vi "Detect change of parameters.vi"(10 "AOL_Globals":T1={"Imaging Protocol"=enum."AOL Z-Stack", "Number of POI"=0, "Number of Miniscans"=0, "Number of Trials"=0, "Number of Cycles "=0, "# Averaged Frames"=0, "Laser power (%)"=0, "Pockels (V)"=0.0, "Acquisition Length (sec)"=0.0, "Fill time (us)"=0.0, "POI Dwell time (us)"=0.0, "Miniscan Dwell time per pixel (us)"=0.0, "PMT 1"=0.0, "PMT 2"=0.0, "Back Apperture (mA)"=0.0, "Frame Size"=0, "Center Frequency"=0.0, "Field of View (um)"=175.0, "Field of View (norm)"=0.0, "DwellTime (us)"=0.0, "Ref Dwell Time (us)"=0.0, "Wavelength (nm)"=0.0, "Zoom"=0.0, "AOL Z"=0.0, "AOL Mode"=enum."Raster", "GridXY"=0.0, "GridZ"=0.0, "TriggerPeriod (sec)"=0.0, "Number of Pixels in Miniscan"=0, "Experiment folder path"=path "", "X centre"=0.0, "Y centre"=0.0, "Angle (degrees)"=0.0, "Angle Xs (degrees)"=0.0, "Angle Ys (degrees)"=0.0, "Plane Mode"=0, "Threshold"=[], "Regenerate Chirps"=FALSE, "Rectangle ROI length (pixels)"=0, "Rectangle ROI height (pixels)"=0, "AOD fill"=4900, "StartupDelay"=0, "Samples Wait after Trigger"=5080, "Slip Cycle"=600000, "Add Cycle"=TRUE, "Functional Mode"=enum."Point", "Z Start"=0.0, "Z Stop"=0.0, "# Planes"=0, "Total Pixels"=0, "Variable Miniscan Pixels"=[], "Use Variable Length"=FALSE, "Use Variable Resolution"=FALSE, "Laser power (%) at Z Start"=0, "Laser power (%) at Z Stop"=0, "Ref Z Step"=0} {"Angle Ys (degrees)" format="%#.6g"; "Angle Xs (degrees)" format="%#.6g"; "Plane Mode" items=["XY Plane", "XZ Plane", "YZ Plane", "arbitraryplane"]; "Frame Size" items=["100X100"=100, "128X128"=128, "200X200"=200, "256X256"=256, "512X512"=512, "1024x1024"=1024, "2048x2048"=2048]; "Back Apperture (mA)" format="%#.6g"; "Pockels (V)" format="%#.6g"; "PMT 2" format="%#.6g"; "PMT 1" format="%#.6g"; "Angle (degrees)" format="%#.6g"; "POI Dwell time (us)" format="%#.6g"}, 11 "ZStack":cluster{"Zstart":dbl, "Zstop":dbl, "Zstep":dbl}) -> (3 "Setup has changed":bool)   [LabVIEW 2020]
uses:
  Typedefs/Controls/AOL_Globals.ctl
  Typedefs/Imaging Protocols enum.ctl
  Typedefs/Frame Size.ctl
  Typedefs/AOL modes.ctl
  Typedefs/Plane Mode.ctl
  Typedefs/Functional Mode.ctl
  Typedefs/Chirps regen checked params.ctl
  Global Variables/General Globals.vi
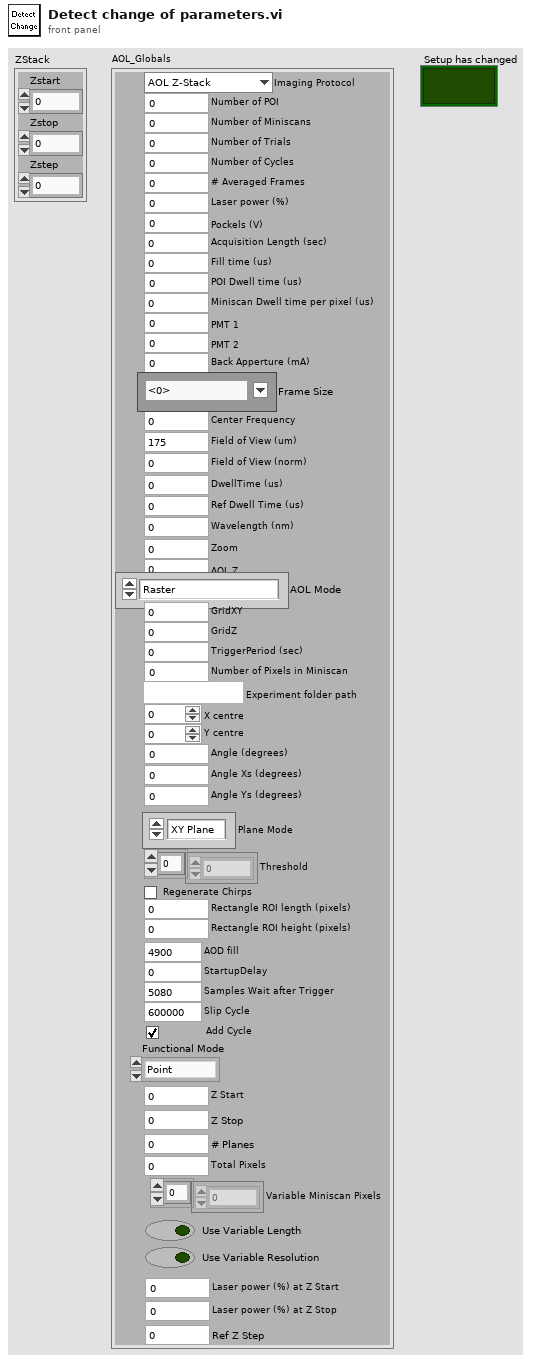
[diagram p1: front panel]
types:
  T1 = typedef "AOL_Globals.ctl" = cluster{"Imaging Protocol":T2, "Number of POI":u16, "Number of Miniscans":u16, "Number of Trials":u16, "Number of Cycles ":u64, "# Averaged Frames":u16, "Laser power (%)":u8, "Pockels (V)":dbl, "Acquisition Length (sec)":dbl, "Fill time (us)":dbl, "POI Dwell time (us)":dbl, "Miniscan Dwell time per pixel (us)":dbl, "PMT 1":dbl, "PMT 2":dbl, "Back Apperture (mA)":dbl, "Frame Size":T3, "Center Frequency":dbl, "Field of View (um)":dbl, "Field of View (norm)":dbl, "DwellTime (us)":dbl, "Ref Dwell Time (us)":dbl, "Wavelength (nm)":dbl, "Zoom":dbl, "AOL Z":dbl, "AOL Mode":T4, "GridXY":dbl, "GridZ":dbl, "TriggerPeriod (sec)":dbl, "Number of Pixels in Miniscan":u16, "Experiment folder path":path, "X centre":dbl, "Y centre":dbl, "Angle (degrees)":dbl, "Angle Xs (degrees)":dbl, "Angle Ys (degrees)":dbl, "Plane Mode":T5, "Threshold":u16[], "Regenerate Chirps":bool, "Rectangle ROI length (pixels)":u16, "Rectangle ROI height (pixels)":u16, "AOD fill":u16, "StartupDelay":i32, "Samples Wait after Trigger":u16, "Slip Cycle":u32, "Add Cycle":bool, "Functional Mode":T6, "Z Start":dbl, "Z Stop":dbl, "# Planes":i32, "Total Pixels":i32, "Variable Miniscan Pixels":u16[], "Use Variable Length":bool, "Use Variable Resolution":bool, "Laser power (%) at Z Start":u8, "Laser power (%) at Z Stop":u8, "Ref Z Step":i8}
  T2 = typedef "Imaging Protocols enum.ctl" = enum16{"AOL Z-Stack", "Motor Z Stack", "Parameter Sweep", "Functional Acquisition", "Single Plane Acquisition", "Volume Acquisition", "Live Imaging", "Live Plane Imaging", "Live Volume Imaging"}
  T3 = typedef "Frame Size.ctl" = u16
  T4 = typedef "AOL modes.ctl" = enum16{"Raster", "Structural", "Pointing", "Mini Scan", "Alignment"}
  T5 = typedef "Plane Mode.ctl" = u16
  T6 = typedef "Functional Mode.ctl" = enum16{"Point", "Line", "Patch", "Plane", "Volume"}
  T7 = typedef "Chirps regen checked params.ctl" = cluster{"Laser power (%)":u8, "Field of View":dbl, "Frame Size":T3, "AOL Z":dbl, "DwellTime (us)":dbl, "Zoom":dbl, "Number of POI":u16, "Number of Miniscans":u16, "POI Dwell time (us)":dbl, "Miniscan Dwell time per pixel (us)":dbl, "Number of Pixels in Miniscan":u16, "X centre":dbl, "Y centre":dbl, "Wavelength (nm)":dbl, "Angle (degrees)":dbl, "Angle Xs (degrees)":dbl, "Angle Ys (degrees)":dbl, "Plane Mode":T5, "Regenerate Chirps":bool, "Ref Z Step":i8}
  T8 = cluster{"ZStack":cluster{"Zstart":dbl, "Zstop":dbl, "Zstep":dbl}, "Checked parameters":T7}
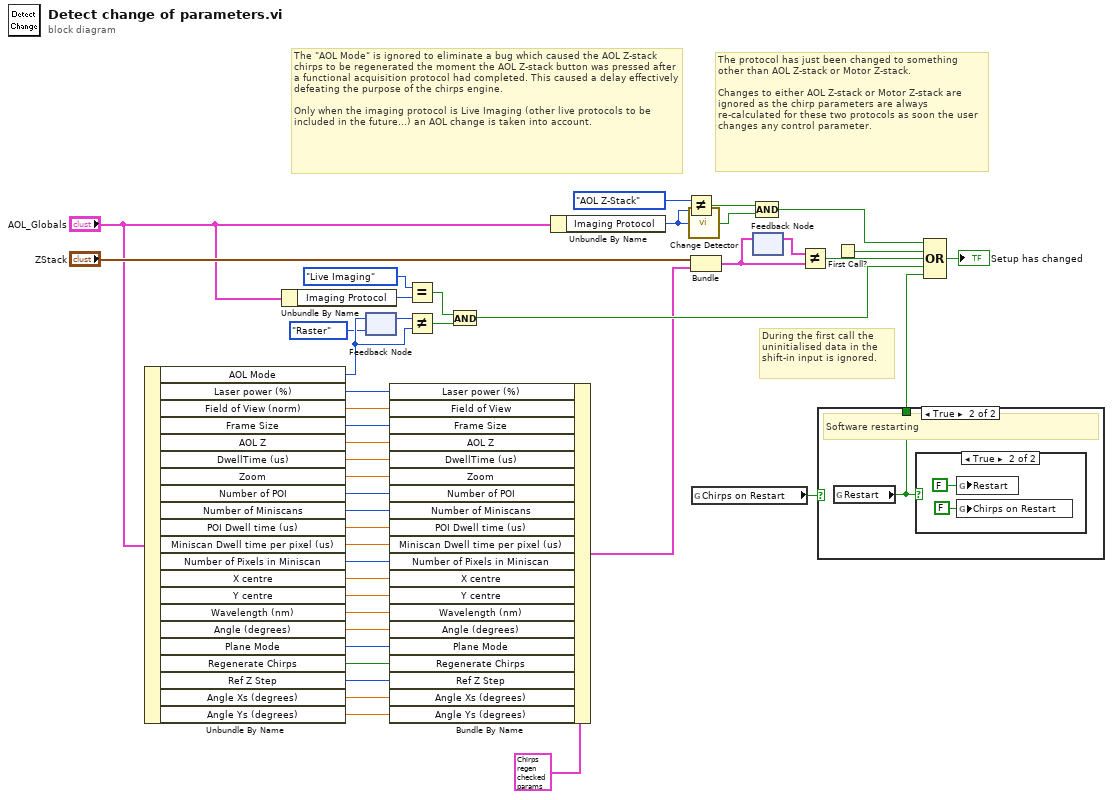
[diagram p0: block diagram]
diagram:
  # "The \"AOL Mode\" is ignored to eliminate a bug which caused the AOL Z-stack chirps to be regenerated the moment the AOL Z-stack button was pressed after a functional acquisition protocol had completed. This caused a delay effectively defeating the purpose of the chirps engine.\n\nOnly when the imaging protocol is Live Imaging (other live protocols to be included in the future...) an AOL change is taken into account."
  # "The protocol has just been changed to something other than AOL Z-stack or Motor Z-stack.\n\nChanges to either AOL Z-stack or Motor Z-stack are ignored as the chirp parameters are always re-calculated for these two protocols as soon the user changes any control parameter."
  # "During the first call the uninitialised data in the shift-in input is ignored."
  n1 = Unbundle By Name("AOL_Globals") -> ("AOL Mode"=w16:T4, "Laser power (%)"=w35:u8, "Field of View (norm)"=w34:dbl, "Frame Size"=w33:T3, "AOL Z"=w32:dbl, "DwellTime (us)"=w31:dbl, "Zoom"=w30:dbl, "Number of POI"=w29:u16, "Number of Miniscans"=w28:u16, "POI Dwell time (us)"=w27:dbl, "Miniscan Dwell time per pixel (us)"=w26:dbl, "Number of Pixels in Miniscan"=w25:u16, "X centre"=w24:dbl, "Y centre"=w23:dbl, "Wavelength (nm)"=w22:dbl, "Angle (degrees)"=w21:dbl, "Plane Mode"=w20:T5, "Regenerate Chirps"=w19:bool, "Ref Z Step"=w3:i8, "Angle Xs (degrees)"=w2:dbl, "Angle Ys (degrees)"=w1:dbl)
  n2 = Unbundle By Name("AOL_Globals") -> ("Imaging Protocol"=w15:T2)
  n3 = feedback-in #1(w16) -> ()
  n4 = feedback #1(AOL_modes."Raster" ("AOL Mode")) -> (w18:T4)
  n5 = Bundle By Name(cluster=T7 {"Laser power (%)"=0, "Field of View"=0.0, "Frame Size"=0, "AOL Z"=0.0, "DwellTime (us)"=0.0, "Zoom"=0.0, "Number of POI"=0, "Number of Miniscans"=0, "POI Dwell time (us)"=0.0, "Miniscan Dwell time per pixel (us)"=0.0, "Number of Pixels in Miniscan"=0, "X centre"=0.0, "Y centre"=0.0, "Wavelength (nm)"=0.0, "Angle (degrees)"=0.0, "Angle Xs (degrees)"=0.0, "Angle Ys (degrees)"=0.0, "Plane Mode"=0, "Regenerate Chirps"=FALSE, "Ref Z Step"=0} ("Checked parameters"), "Laser power (%)"=w35, "Field of View"=w34, "Frame Size"=w33, "AOL Z"=w32, "DwellTime (us)"=w31, "Zoom"=w30, "Number of POI"=w29, "Number of Miniscans"=w28, "POI Dwell time (us)"=w27, "Miniscan Dwell time per pixel (us)"=w26, "Number of Pixels in Miniscan"=w25, "X centre"=w24, "Y centre"=w23, "Wavelength (nm)"=w22, "Angle (degrees)"=w21, "Plane Mode"=w20, "Regenerate Chirps"=w19, "Ref Z Step"=w3, "Angle Xs (degrees)"=w2, "Angle Ys (degrees)"=w1) -> (w8:T7)
  n6 = Equal?(x=Imaging_Protocols_enum."Live Imaging", y=w15) -> (x = y?=w14:bool)
  n7 = Not Equal?(x=w18, y=w16) -> (x != y?=w17:bool)
  n8 = And(x=w14, y=w17) -> (x .and. y?=w11:bool)
  n9 = Unbundle By Name("AOL_Globals") -> ("Imaging Protocol"=w39:T2)
  n10 = Not Equal?(x=Imaging_Protocols_enum."AOL Z-Stack", y=w39) -> (x != y?=w40:bool)
  n11 = call <userlib>:"Change Detector.vi"("Value"=w39) -> ("Changed?"=w37:bool)
  n12 = Bundle("ZStack"="ZStack", "Checked parameters"=w8) -> (w12:T8)  [unwired: 1 in]
  n13 = global read "General Globals.vi" "Chirps on Restart"() -> (w5:bool)
  n14 = feedback-in #2(w12) -> ()
  n15 = feedback #2() -> (w13:T8)  [unwired: 1 in]
  n16 = Compound Arithmetic op=AND(w40, w37) -> (w36:bool)
  n17 = Not Equal?(x=w13, y=w12) -> (x != y?=w43:bool)
  n18 = case shown="True" w5 {
    tunnel: [_ w45] -> w6
    frame False {
    }
    frame True {
      # "Software restarting"
      n19 = global read "General Globals.vi" "Restart"() -> (w45:bool)
      n20 = case shown="True" w45 {
        frame False {
        }
        frame True {
          n21 = global write "General Globals.vi" "Restart"(FALSE ("Restart")) -> ()
          n22 = global write "General Globals.vi" "Chirps on Restart"(FALSE ("Restart")) -> ()
        }
      }
    }
  }
  n23 = First Call?() -> (First Call?: T/F=w44:bool)
  n24 = Compound Arithmetic op=OR(w36, w44, w43, w11, w6) -> (→"Setup has changed":bool)
